vi "Add States to Routing and Faulting Custom Device.vi"() -> ()   [LabVIEW 2019]
uses:
  NationalInstruments.VeriStand.SystemDefinitionAPI
  SLSC Switch Examples.lvlib
  <vilib>/addons/VeriStand Custom Device Scripting APIs/Routing and Faulting/Scripting/Routing and Faulting Scripting.lvlib
panel:
  in  "Channel Name":string="Window Up"
  in  "New State Configuration":T1={"Name"="My New State", "Description"="new description", "Value"=10.0, "Connection List"=[{"Module Path"="Targets/Controller/Hardware/SLSC/SLSC Chassis/Modules/Slot 2 (SLSC Switch)", "Source"="DUT_Ch6", "Destination"="LOAD_Ch6"}]}
  in  "Output System Definition File":path=path "System Definition Files/Scripted Routing and Faulting.nivssdf"
  in  "Input System Definition File (Preconfigured with a Routing and Faulting custom device)":path=path "System Definition Files/Base with Routing and Faulting.nivssdf"
  # "Overview: Demonstrates using the Routing and Faulting scripting API to add a routing channel state to the custom device. \n\nInstructions:\n1. Use one of the SLSC Switch scripting examples (Configure Modules ...) to script one SLSC Switch custom devices into a system definition file.\n2. Use the Configure Routing and Faulting Custom Device example to add a configured Routing and Faulting custom device to the system definition from step 1.\n3. Browse to a path to save the system definition file as the output Output System Definition File.  This may be the same as the input file.\n4. Run the VI and verify its results."
  # "System Definition Files"
  # "Routing and Faulting Custom Device Configuration"
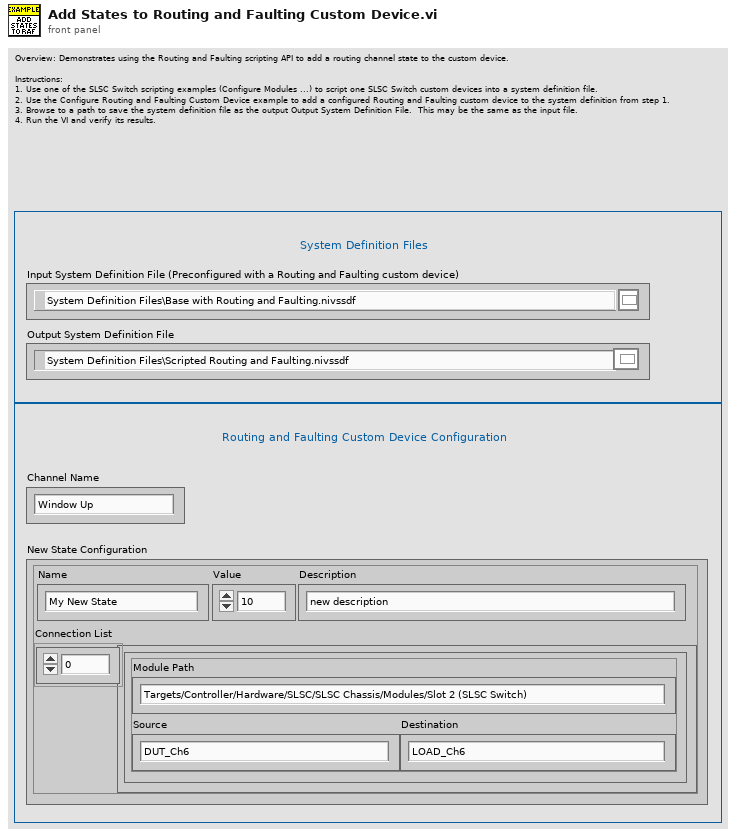
[diagram p1: front panel]
types:
  T1 = cluster{"Name":string, "Description":string, "Value":dbl, "Connection List":cluster{"Module Path":string, "Source":string, "Destination":string}[]}
  T2 = typedef "Custom Device API.lvlib/Custom Device Item Ref.ctl" = u64
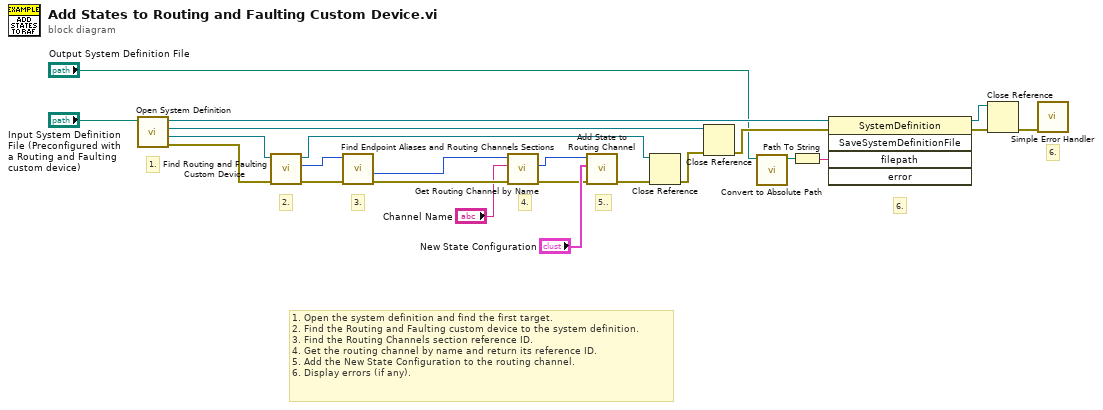
[diagram p0: block diagram]
diagram:
  # "5.."
  # "4."
  # "3."
  # "2."
  # "6."
  # "6."
  # "8."
  # "1."
  # "1. Open the system definition and find the first target.\n2. Find the Routing and Faulting custom device to the system definition.\n3. Find the Routing Channels section reference ID.\n4. Get the routing channel by name and return its reference ID.\n5. Add the New State Configuration to the routing channel.\n6. Display errors (if any)."
  n1 = call "Open System Definition.vi"("System Definition File"="Input System Definition File (Preconfigured with a Routing and Faulting custom device)") -> ("error out"=w9:errorcluster, "Target Refnum"=w13:refnum<k24>, "Root Refnum"=w19:refnum<k24>, "System Definition Refnum"=w23:refnum<k24>)  [unwired: 7 in]
  n2 = call <vilib>:"Find Routing and Faulting Custom Device.vi"("error in"=w9, "target in"=w13) -> ("error out"=w11:errorcluster, "routing and faulting custom device"=w12:T2, "target out"=w10:refnum<k24>)  [unwired: 7 in]
  n3 = call <vilib>:"Find Endpoint Aliases and Routing Channels Sections.vi"("error in"=w11, "routing and faulting custom device in"=w12) -> ("error out"=w4:errorcluster, "routing channels"=w5:T2)  [unwired: 6 in, 2 out]
  n4 = call <vilib>:"Get Routing Channel by Name.vi"("error in"=w4, "channel name"="Channel Name", "routing channels in"=w5) -> ("error out"=w2:errorcluster, "routing channel"=w6:T2)  [unwired: 6 in, 1 out]
  n5 = call <vilib>:"Add State to Routing Channel.vi"("error in"=w2, "state and connections"="New State Configuration", "routing channel in"=w6) -> ("error out"=w7:errorcluster)  [unwired: 7 in, 1 out]
  n6 = Close Reference(reference=w10, error in (no error)=w7) -> (error out=w16:errorcluster)
  n7 = Close Reference(reference=w19, error in (no error)=w16) -> (error out=w18:errorcluster)
  n8 = call "Convert to Absolute Path.vi"("System Definition File"="Output System Definition File") -> ("Absolute Path"=w1:path)  [unwired: 10 in]
  n9 = Path To String(path=w1) -> (string=w22:string)
  n10 = invoke class="SystemDefinition" method="SaveSystemDefinitionFile"(reference=w23, error in=w18, "filepath"=w22) -> (reference out=w20:refnum<k24>, error out=w21:errorcluster)  [unwired: 2 in, 3 out]
  n11 = Close Reference(reference=w20, error in (no error)=w21) -> (error out=w15:errorcluster)
  n12 = call <vilib>:"Simple Error Handler.vi"("error in (no error)"=w15) -> ()  [unwired: 1 in, 8 out]
